vi "Final.vi"() -> ()   [LabVIEW 2023]
uses:
  <vilib>/DAQmx/read.llb/DAQmx Read (Digital 1D Bool 1Chan 1Samp).vi
  <vilib>/DAQmx/read.llb/DAQmx Read (Analog DBL 1Chan 1Samp).vi
  <vilib>/DAQmx/read.llb/DAQmx Read (Digital Bool 1Line 1Point).vi
  <vilib>/DAQmx/write.llb/DAQmx Write (Digital Bool 1Line 1Point).vi
  <vilib>/DAQmx/create/channels.llb/DAQmx Create Channel (DO-Digital Output).vi
  <vilib>/DAQmx/create/channels.llb/DAQmx Create Channel (DI-Digital Input).vi
  <vilib>/DAQmx/create/channels.llb/DAQmx Create Channel (AI-Voltage-Basic).vi
  <vilib>/DAQmx/miscellaneous.llb/DAQmx Fill In Error Info.vi
panel:
  in  "stop 2":bool
  in  "stop":bool
  out "x-y":u32
  out "Meter":dbl(knob) scale=0.0..500.0
  out "Thermometer":dbl(slide) scale=0.0..100.0
  out "Cry":bool
  in  "Fan":tag
  in  "Temperatue Sensor":tag
  in  "Speed 2":tag
  in  "Speed 1":tag
  in  "Presence":tag
  in  "Motor":tag
  in  "Sound Sensor":tag
  in  "Rain Sensor":tag
  in  "Buzzer":tag
  out "Wet":bool
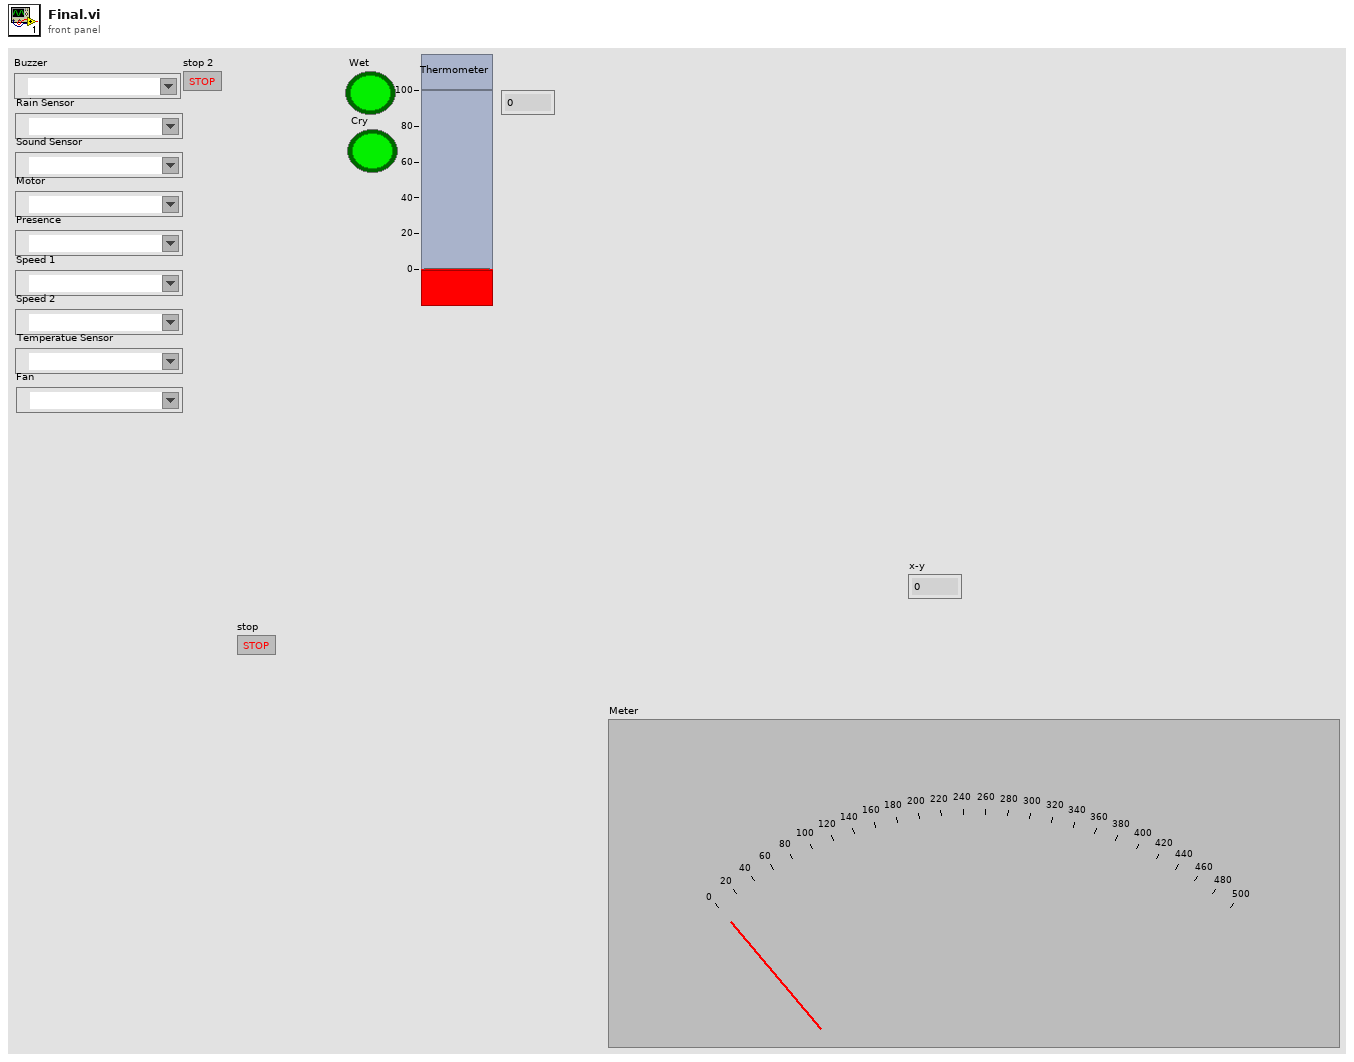
[diagram p1: front panel]
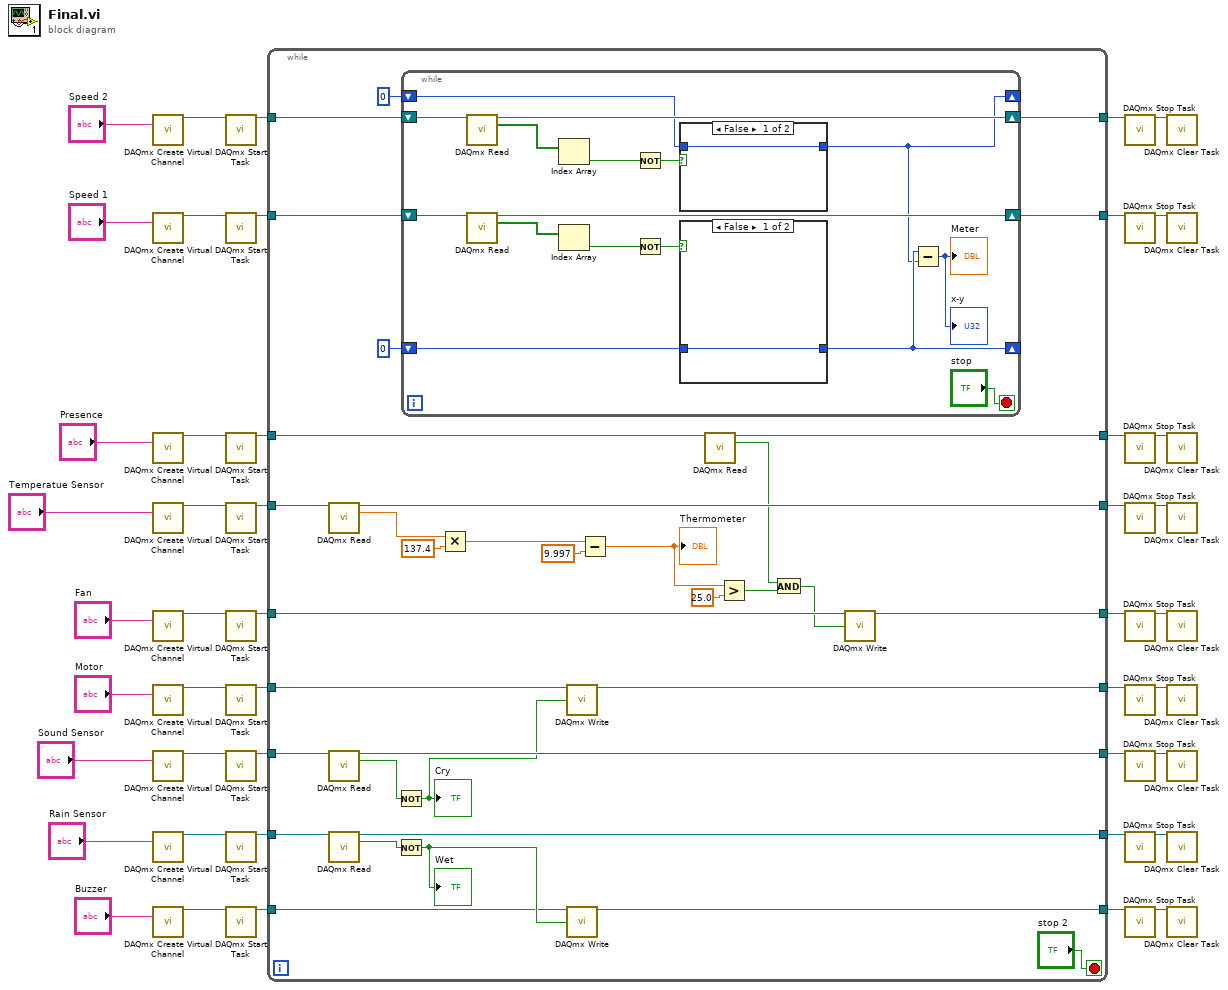
[diagram p0: block diagram]
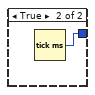
[diagram p2: hidden frame]
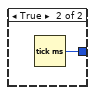
[diagram p3: hidden frame]
diagram:
  n1 = call-poly <vilib>:"DAQmx Create Virtual Channel.vi"("lines"="Speed 2") -> ("task out"=w22:refnum<k21>)  [unwired: 13 in, 1 out]
  n2 = call-poly <vilib>:"DAQmx Create Virtual Channel.vi"("lines"="Speed 1") -> ("task out"=w23:refnum<k21>)  [unwired: 13 in, 1 out]
  n3 = call-poly <vilib>:"DAQmx Create Virtual Channel.vi"("lines"="Presence") -> ("task out"=w28:refnum<k21>)  [unwired: 13 in, 1 out]
  n4 = call-poly <vilib>:"DAQmx Create Virtual Channel.vi"("physical channels"="Temperatue Sensor") -> ("task out"=w25:refnum<k21>)  [unwired: 13 in, 1 out]
  n5 = call-poly <vilib>:"DAQmx Create Virtual Channel.vi"("lines"="Fan") -> ("task out"=w24:refnum<k21>)  [unwired: 13 in, 1 out]
  n6 = call-poly <vilib>:"DAQmx Create Virtual Channel.vi"("lines"="Motor") -> ("task out"=w27:refnum<k21>)  [unwired: 13 in, 1 out]
  n7 = call-poly <vilib>:"DAQmx Create Virtual Channel.vi"("lines"="Sound Sensor") -> ("task out"=w26:refnum<k21>)  [unwired: 13 in, 1 out]
  n8 = call-poly <vilib>:"DAQmx Create Virtual Channel.vi"("lines"="Rain Sensor") -> ("task out"=w37:refnum<k21>)  [unwired: 13 in, 1 out]
  n9 = call-poly <vilib>:"DAQmx Create Virtual Channel.vi"("lines"="Buzzer") -> ("task out"=w39:refnum<k21>)  [unwired: 13 in, 1 out]
  n10 = call <vilib>:"DAQmx Start Task.vi"("task/channels in"=w22) -> ("task out"=w10:refnum<k21>)  [unwired: 13 in, 1 out]
  n11 = call <vilib>:"DAQmx Start Task.vi"("task/channels in"=w23) -> ("task out"=w11:refnum<k21>)  [unwired: 13 in, 1 out]
  n12 = call <vilib>:"DAQmx Start Task.vi"("task/channels in"=w28) -> ("task out"=w18:refnum<k21>)  [unwired: 13 in, 1 out]
  n13 = call <vilib>:"DAQmx Start Task.vi"("task/channels in"=w25) -> ("task out"=w17:refnum<k21>)  [unwired: 13 in, 1 out]
  n14 = call <vilib>:"DAQmx Start Task.vi"("task/channels in"=w24) -> ("task out"=w20:refnum<k21>)  [unwired: 13 in, 1 out]
  n15 = call <vilib>:"DAQmx Start Task.vi"("task/channels in"=w27) -> ("task out"=w21:refnum<k21>)  [unwired: 13 in, 1 out]
  n16 = call <vilib>:"DAQmx Start Task.vi"("task/channels in"=w26) -> ("task out"=w19:refnum<k21>)  [unwired: 13 in, 1 out]
  n17 = call <vilib>:"DAQmx Start Task.vi"("task/channels in"=w37) -> ("task out"=w36:refnum<k21>)  [unwired: 13 in, 1 out]
  n18 = call <vilib>:"DAQmx Start Task.vi"("task/channels in"=w39) -> ("task out"=w38:refnum<k21>)  [unwired: 13 in, 1 out]
  n19 = while {
    tunnel: [w77] -> w43
    tunnel: [w76] -> w41
    tunnel: w38 -> [w75]
    tunnel: w36 -> [w74]
    tunnel: w21 -> [w73]
    tunnel: w20 -> [w72]
    tunnel: w19 -> [w71]
    tunnel: w18 -> [w70]
    tunnel: w17 -> [w69]
    tunnel: [w68] -> w16
    tunnel: [w67] -> w15
    tunnel: [w66] -> w14
    tunnel: [w65] -> w13
    tunnel: [w64] -> w12
    tunnel: w11 -> [w50]
    tunnel: w10 -> [w49]
    tunnel: [w48] -> w9
    tunnel: [w47] -> w8
    stop <- "stop 2" stop-if-true
    n20 = call-poly <vilib>:"DAQmx Read.vi"("task/channels in"=w69) -> ("task out"=w65:refnum<k21>, "data"=w58:dbl)  [unwired: 12 in, 1 out]
    n21 = call-poly <vilib>:"DAQmx Read.vi"("task/channels in"=w71) -> ("task out"=w68:refnum<k21>, "data"=w63:bool)  [unwired: 12 in, 1 out]
    n22 = call-poly <vilib>:"DAQmx Read.vi"("task/channels in"=w74) -> ("task out"=w77:refnum<k21>, "data"=w79:bool)  [unwired: 12 in, 1 out]
    n23 = Not(x=w63) -> (.not. x?=w62:bool)
    "Cry" <- w62
    n24 = Not(x=w79) -> (.not. x?=w78:bool)
    "Wet" <- w78
    n25 = while {
      shift-right: [w94] -> w48
      shift-left: w50 -> [w95]
      shift-right: [w92] -> w47
      shift-left: w49 -> [w93]
      shift-right: [w85] -> _
      shift-left: u32 0 ("millisecond timer value") -> [w82]
      shift-right: [w84] -> _
      shift-left: u32 0 ("millisecond timer value") -> [w81]
      stop <- "stop" stop-if-true
      n26 = call-poly <vilib>:"DAQmx Read.vi"("task/channels in"=w93) -> ("task out"=w92:refnum<k21>, "data"=w89:bool[])  [unwired: 12 in, 1 out]
      n27 = call-poly <vilib>:"DAQmx Read.vi"("task/channels in"=w95) -> ("task out"=w94:refnum<k21>, "data"=w90:bool[])  [unwired: 12 in, 1 out]
      n28 = Index Array(array=w89) -> (element=w87:bool)  [unwired: 1 in]
      n29 = Index Array(array=w90) -> (element=w88:bool)  [unwired: 1 in]
      n30 = Not(x=w87) -> (.not. x?=w83:bool)
      n31 = Not(x=w88) -> (.not. x?=w86:bool)
      n32 = case shown="False" w83 {
        tunnel: [w96 w97] -> w84
        tunnel: w81 -> [w96 _]
        frame False {
        }
        frame True {
          n33 = Tick Count (ms)() -> (millisecond timer value=w97:u32)
        }
      }
      n34 = case shown="False" w86 {
        tunnel: [w98 w99] -> w85
        tunnel: w82 -> [w98 _]
        frame False {
        }
        frame True {
          n35 = Tick Count (ms)() -> (millisecond timer value=w99:u32)
        }
      }
      n36 = Subtract(x=w85, y=w84) -> (x-y=→"x-y" →"Meter":u32)
    }
    n37 = Multiply(x=w58, y=137.4) -> (x*y=w60:dbl)
    n38 = call-poly <vilib>:"DAQmx Write.vi"("task/channels in"=w73, "data"=w62) -> ("task out"=w67:refnum<k21>)  [unwired: 11 in, 2 out]
    n39 = call-poly <vilib>:"DAQmx Write.vi"("task/channels in"=w75, "data"=w78) -> ("task out"=w76:refnum<k21>)  [unwired: 11 in, 2 out]
    n40 = Subtract(x=w60, y=9.997) -> (x-y=w57:dbl)
    "Thermometer" <- w57
    n41 = call-poly <vilib>:"DAQmx Read.vi"("task/channels in"=w70) -> ("task out"=w66:refnum<k21>, "data"=w55:bool)  [unwired: 12 in, 1 out]
    n42 = Greater?(x=w57, y=25.0) -> (0:w54:bool)
    n43 = And(x=w55, y=w54) -> (x .and. y?=w53:bool)
    n44 = call-poly <vilib>:"DAQmx Write.vi"("task/channels in"=w72, "data"=w53) -> ("task out"=w64:refnum<k21>)  [unwired: 11 in, 2 out]
  }
  n45 = call <vilib>:"DAQmx Stop Task.vi"("task/channels in"=w8) -> ("task out"=w1:refnum<k21>)  [unwired: 13 in, 1 out]
  n46 = call <vilib>:"DAQmx Stop Task.vi"("task/channels in"=w9) -> ("task out"=w2:refnum<k21>)  [unwired: 13 in, 1 out]
  n47 = call <vilib>:"DAQmx Stop Task.vi"("task/channels in"=w14) -> ("task out"=w5:refnum<k21>)  [unwired: 13 in, 1 out]
  n48 = call <vilib>:"DAQmx Stop Task.vi"("task/channels in"=w13) -> ("task out"=w4:refnum<k21>)  [unwired: 13 in, 1 out]
  n49 = call <vilib>:"DAQmx Stop Task.vi"("task/channels in"=w12) -> ("task out"=w3:refnum<k21>)  [unwired: 13 in, 1 out]
  n50 = call <vilib>:"DAQmx Stop Task.vi"("task/channels in"=w15) -> ("task out"=w6:refnum<k21>)  [unwired: 13 in, 1 out]
  n51 = call <vilib>:"DAQmx Stop Task.vi"("task/channels in"=w16) -> ("task out"=w7:refnum<k21>)  [unwired: 13 in, 1 out]
  n52 = call <vilib>:"DAQmx Stop Task.vi"("task/channels in"=w43) -> ("task out"=w42:refnum<k21>)  [unwired: 13 in, 1 out]
  n53 = call <vilib>:"DAQmx Stop Task.vi"("task/channels in"=w41) -> ("task out"=w40:refnum<k21>)  [unwired: 13 in, 1 out]
  n54 = call <vilib>:"DAQmx Clear Task.vi"("task in"=w1) -> ()  [unwired: 14 in, 1 out]
  n55 = call <vilib>:"DAQmx Clear Task.vi"("task in"=w2) -> ()  [unwired: 14 in, 1 out]
  n56 = call <vilib>:"DAQmx Clear Task.vi"("task in"=w5) -> ()  [unwired: 14 in, 1 out]
  n57 = call <vilib>:"DAQmx Clear Task.vi"("task in"=w4) -> ()  [unwired: 14 in, 1 out]
  n58 = call <vilib>:"DAQmx Clear Task.vi"("task in"=w3) -> ()  [unwired: 14 in, 1 out]
  n59 = call <vilib>:"DAQmx Clear Task.vi"("task in"=w6) -> ()  [unwired: 14 in, 1 out]
  n60 = call <vilib>:"DAQmx Clear Task.vi"("task in"=w7) -> ()  [unwired: 14 in, 1 out]
  n61 = call <vilib>:"DAQmx Clear Task.vi"("task in"=w42) -> ()  [unwired: 14 in, 1 out]
  n62 = call <vilib>:"DAQmx Clear Task.vi"("task in"=w40) -> ()  [unwired: 14 in, 1 out]
